vi "5000_CPU_configure.vi"() -> ()   [LabVIEW 2010]
panel:
  out "String including Checksum":string
  out "Timed out":bool
  out "Serial Error":bool
  in  "Port Name":string="MainNetwork"
  in  "Baud Rate (9600)":u16(ring)=3 items=["1200 bps", "2400 bps", "4800 bps", "9600 bps", "19.2 kbps", "38.4 kbps", "57.6 kbps", "115.2 kbps"]
  out "Reply":string
  out "String to send":string
  # "To Configure the ADAM 5000 CPU\n\n1) First Set the node id switches to the desired module address that you would like the  ADAM 5000 to have\n\n2) Then power up the 5000 with the INIT* conected to zero volts.\n\n3) Run this Vi to set the Baud rate etc to the desired values.\n\n4) You should get a reply  like  !78/r  where 78 is the address you have set with the switches in hex\n\n5) Now power down the 5000 and disconnect the wire to  INIT* \n\n6) Power the  5000 back up and you should be able to talk to it using the address you have set in (1)"
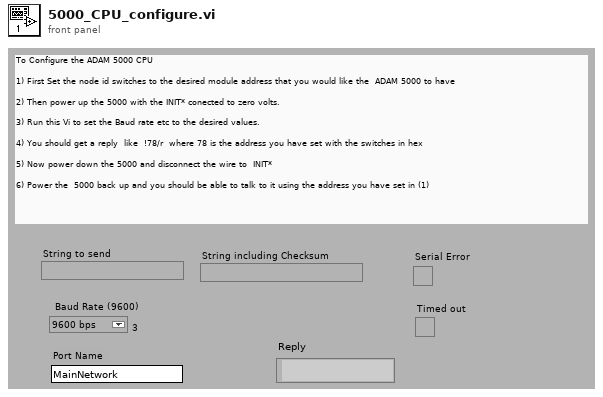
[diagram p1: front panel]
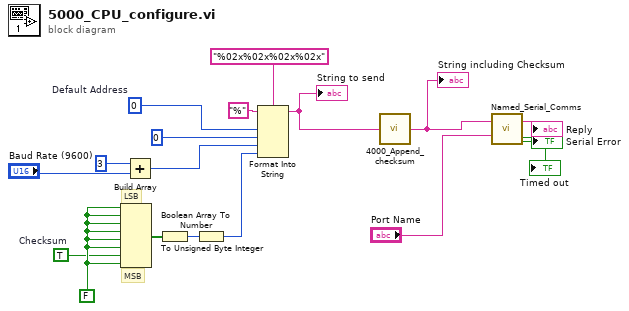
[diagram p0: block diagram]
diagram:
  w2 = u8 0  # Default Address
  w3 = TRUE  # Checksum
  w12 = FALSE
  # "MSB"
  # "LSB"
  n1 = Build Array(w12, w12, w12, w12, w12, w12, w3, w12) -> (w16:bool[])
  n2 = Add(x=u16 3, y="Baud Rate (9600)") -> (x+y=w8:u16)
  n3 = Boolean Array To Number(Boolean array=w16) -> (number=w15:u32)
  n4 = To Unsigned Byte Integer(number=w15) -> (unsigned 8bit integer=w7:u8)
  n5 = Format Into String(format string="%02x%02x%02x%02x", initial string="%", w2, u8 0 ("New Address"), w8, w7) -> (resulting string=w14:string)  [unwired: 1 in, 1 out]
  "String to send" <- w14
  n6 = call "4000_Append_checksum.vi"("ADAM command"=w14) -> ("ADAM string to send"=w1:string)
  "String including Checksum" <- w1
  n7 = call "Named_Serial_Comms.vi"("Write String"=w1, "Port Name"="Port Name") -> ("Read"=→"Reply":string, "Timed out"=→"Timed out":bool, "Serial Error"=→"Serial Error":bool)  [unwired: 10 in, 1 out]
